vi "write_TIFF_single_page.vi"(6 "description":string, 8 "error in (no error)":errorcluster, 9 "force format?":T1, 10 "data":dbl[][](array[numeric]), 11 "path in":path) -> (0 "error out":errorcluster, 3 "path out":path)   [LabVIEW 2010, in "TIFFManagement.lvlib"]
uses:
  TIFFManagement.lvlib
  classes/Image/Image/target_format_enum.ctl
  VisualCPP/Release/TIFFManagement.dll
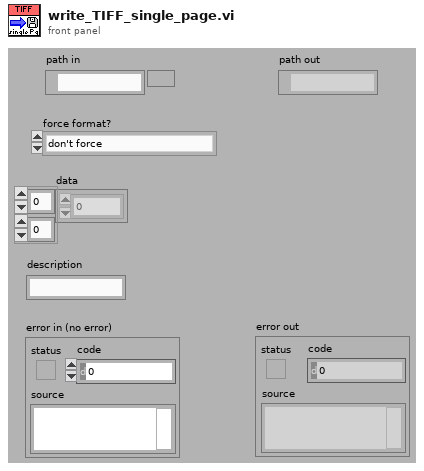
[diagram p1: front panel]
types:
  T1 = typedef "target_format_enum.ctl" = enum16{"don't force", "uint8", "uint16", "int16", "uint32", "int32", "single float"}
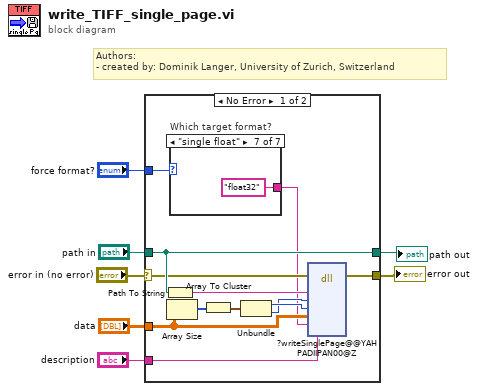
[diagram p0: block diagram]
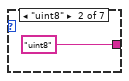
[diagram p3: hidden frame]
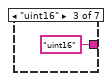
[diagram p4: hidden frame]
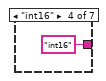
[diagram p5: hidden frame]
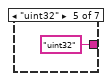
[diagram p6: hidden frame]
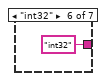
[diagram p7: hidden frame]
diagram:
  # "Authors: \n- created by: Dominik Langer, University of Zurich, Switzerland"
  n1 = case shown="No Error" "error in (no error)" {
    selector: "error in (no error)" -> [w9 w27]
    tunnel: "path in" -> [w15 w26]
    tunnel: [w19 w27] -> w5
    tunnel: [w15 w26] -> w4
    tunnel: "data" -> [w11 _]
    tunnel: "description" -> [w14 _]
    tunnel: "force format?" -> [w10 _]
    frame No Error {
      n2 = Path To String(path=w15) -> (string=w18:string)
      n3 = Array Size(array=w11) -> (size(s)=w17:i32[])
      n4 = case "Which target format?" shown="\"single float\"" w10 {
        tunnel: [_ "uint8" "uint16" "int16" "uint32" "int32" "float32"] -> w8
        frame "don't force", Default {
        }
        frame "uint8" {
        }
        frame "uint16" {
        }
        frame "int16" {
        }
        frame "uint32" {
        }
        frame "int32" {
        }
        frame "single float" {
        }
      }
      n5 = Array To Cluster(array=w17) -> (cluster=w16:cluster{"[0]":i32, "[1]":i32})
      n6 = Unbundle(w16) -> ("[0]"=w13:i32, "[1]"=w12:i32)
      n7 = dll-call lib="C:/helioscan/common/libraries/TIFFManagement/VisualCPP/Release/TIFFManagement.dll" fn="?writeSinglePage@@YAHPADIIPAN00@Z"(error in=w9, "path"=w18, "width"=w12, "height"=w13, "data"=w11, "format"=w8, "description"=w14) -> (error out=w19:errorcluster)  [unwired: 9 in, 1 out]
    }
    frame Error {
    }
  }
  "error out" <- w5
  "path out" <- w4
